vi "SQ Lite Globals.vi"() -> ()   [LabVIEW 2017]
panel:
  in  "Path":path=path "C:/Projects/Labview Projects/LabView2017/Beltwatch/DB/Beltwatch.db"
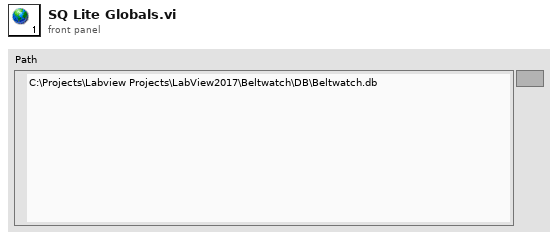
[diagram p1: front panel]
diagram:
